vi "processInputString.vi"(8 "error in (no error)":errorcluster, 10 "stringRead":string, 11 "Model in":refnum<class "Model.lvclass">) -> (0 "error out":errorcluster, 3 "Model out":refnum<class "Model.lvclass">)   [LabVIEW 2013, in "Model.lvclass"]
uses:
  Model.lvclass
  Model.lvclass/Model.ctl
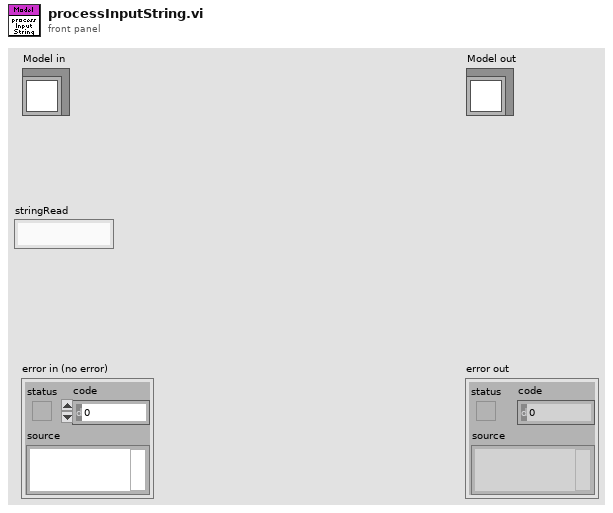
[diagram p1: front panel]
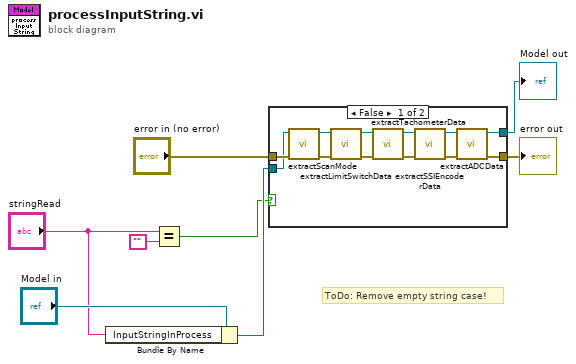
[diagram p0: block diagram]
diagram:
  # "ToDo: Remove empty string case!"
  n1 = Bundle By Name(cluster="Model in", "InputStringInProcess"="stringRead") -> (w6:refnum<class "Model.lvclass">)
  n2 = Equal?(x="stringRead", y="") -> (x = y?=w1:bool)
  n3 = case shown="False" w1 {
    tunnel: "error in (no error)" -> [w16 w22]
    tunnel: w6 -> [w13 w21]
    tunnel: [w10 w22] -> w5
    tunnel: [w9 w21] -> w4
    frame False {
      n4 = call "extractScanMode.vi"("error in (no error)"=w16, "Model in"=w13) -> ("error out"=w15:errorcluster, "Model out"=w17:refnum<class "Model.lvclass">)  [unwired: 8 in]
      n5 = call "extractLimitSwitchData.vi"("error in (no error)"=w15, "Model in"=w17) -> ("error out"=w14:errorcluster, "Model out"=w18:refnum<class "Model.lvclass">)  [unwired: 8 in]
      n6 = call "extractTachometerData.vi"("error in (no error)"=w14, "Model in"=w18) -> ("error out"=w19:errorcluster, "Model out"=w20:refnum<class "Model.lvclass">)  [unwired: 8 in]
      n7 = call "extractSSIEncoderData.vi"("error in (no error)"=w19, "Model in"=w20) -> ("error out"=w11:errorcluster, "Model out"=w12:refnum<class "Model.lvclass">)  [unwired: 8 in]
      n8 = call "extractADCData.vi"("error in (no error)"=w11, "Model in"=w12) -> ("error out"=w10:errorcluster, "Model out"=w9:refnum<class "Model.lvclass">)  [unwired: 8 in]
    }
    frame True {
    }
  }
  "error out" <- w5
  "Model out" <- w4
